vi "Write Digital Port.vi"() -> ()   [LabVIEW 2020]
uses:
  <instrlib>/BDAQ-6104/Public/Data/Write Single Digital Port.vi
  <instrlib>/BDAQ-6104/BDAQ-6104.lvlib
panel:
  in  "Pin State":bool
  in  "Pin Direction":T1(array[cluster])=[{"Pin Number"=enum."Digital Pin 3", "Pin Direction"=TRUE}]
  in  "VISA resource name":refnum<visa-resource-name>
  # "Configures the digital pin as output and writes sets it high."
  # "Input"
  # "Output"
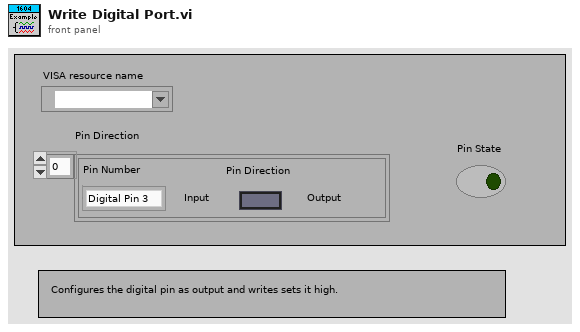
[diagram p1: front panel]
types:
  T1 = cluster{"Pin Number":enum16{"Digital Pin 0", "Digital Pin 1", "Digital Pin 2", "Digital Pin 3"}, "Pin Direction":bool}[]
  T2 = cluster{"Pin Number":enum16{"Digital Pin 0", "Digital Pin 1", "Digital Pin 2", "Digital Pin 3"}, "Pin Direction":bool}
  T3 = enum16{"Digital Pin 0", "Digital Pin 1", "Digital Pin 2", "Digital Pin 3"}
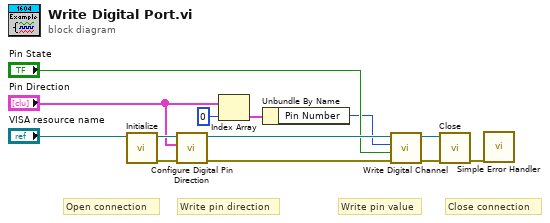
[diagram p0: block diagram]
diagram:
  # "Close connection"
  # "Write pin value"
  # "Write pin direction"
  # "Open connection"
  n1 = call <instrlib>:"Initialize.vi"("VISA resource name"="VISA resource name") -> ("error out"=w8:errorcluster, "VISA resource name out"=w13:refnum<visa-resource-name>)  [unwired: 9 in]
  n2 = call <instrlib>:"Configure Digital Pin Direction.vi"("error in (no error)"=w8, "Pin Direction"="Pin Direction", "VISA resource name"=w13) -> ("error in (no error) 2"=w9:errorcluster, "VISA resource name 2"=w12:refnum<visa-resource-name>)  [unwired: 7 in]
  n3 = Index Array(array="Pin Direction", index=0) -> (element=w2:T2)
  n4 = Unbundle By Name(w2) -> ("Pin Number"=w1:T3)
  n5 = call-poly <instrlib>:"Write Digital Channel.vi"("error in (no error)"=w9, "Pin State"="Pin State", "Pin Number"=w1, "VISA resource name"=w12) -> ("error out"=w10:errorcluster, "VISA resource name out"=w11:refnum<visa-resource-name>)  [unwired: 6 in]
  n6 = call <instrlib>:"Close.vi"("error in (no error)"=w10, "VISA resource name"=w11) -> ("error out"=w5:errorcluster)  [unwired: 9 in]
  n7 = call <vilib>:"Simple Error Handler.vi"("error in (no error)"=w5) -> ()  [unwired: 4 in, 5 out]
